vi "rsscope_core_global.vi"() -> ()   [LabVIEW 2014]
doc: "This Global variable contains driver's:\n- Attributes\n- Range Tables\n- Repeated Capabilities"
uses:
  rsidr_core.llb/type_Input_Format_Attribute.ctl
  rsidr_core.llb/rsscope_rsidr_core.lvlib
  rsidr_core.llb/type_Input_Format_RangeTable.ctl
  rsidr_core.llb/type_Input_Format_RepCap.ctl
panel:
  in  "Repeated Capabilities":T1[](array[typedef])=[{"repCapName"="Channel", "indetifiers"=["CH1", "CH2", "CH3", "CH4", "CHExt"], "cmdValues"=["1", "2", "3", "4", "5"]}, {"repCapName"="Waveform", "indetifiers"=["W0", "W1", "W2", "W3"], "cmdValues"=["1", "1", "2", "3"]}, {"repCapName"="Trigger", "indetifiers"=["TrigA", "TrigB", "TrigR"], "cmdValues"=["1", "2", "3"]}, {"repCapName"="Cursor", "indetifiers"=["C1", "C2", "C3", "C4"], "cmdValues"=["1", "2", "3", "4"]}, {"repCapName"="CPosition", "indetifiers"=["P1", "P2"], "cmdValues"=["1", "2"]}, {"repCapName"="TriggerSource", "indetifiers"=["TsCH1", "TsCH2", "TsCH3", "TsCH4", "TsExt", "TsLine", "TsZ1V1", "TsZ1V2", "TsZ1V3", "TsZ1V4", "TsZ1I1", "TsZ1I2", "TsZ1I3", "TsZ1I4", "TsZ2V1", "TsZ2V2", "TsZ2V3", "TsZ2V4", "TsZ2I1", "TsZ2I2", "TsZ2I3", "TsZ2I4", "TsDiff1", "TsDiff2", "TsCommon1", "TsCommon2"], "cmdValues"=["1", "2", "3", "4", "5", "10", "12", "13", "14", "15", "16", "17", "18", "19", "20", "21", "22", "23", "24", "25", "26", "27", "28", "29", "30", "31"]}, {"repCapName"="TriggerType", "indetifiers"=["Edge", "Width", "Runt", "Glitch", "Window", "Timeout", "Interval", "Slew", "Data2Clock", "Pattern", "External", "T11", "T12", "NFC", "TV", "CDR"], "cmdValues"=["1", "3", "4", "2", "5", "6", "7", "8", "9", "10", "11", "12", "14", "15", "16", "17"]}, {"repCapName"="Measurement", "indetifiers"=["Meas1", "Meas2", "Meas3", "Meas4", "Meas5", "Meas6", "Meas7", "Meas8", "Meas9", "Meas10"], "cmdValues"=["1", "2", "3", "4", "5", "6", "7", "8", "9", "10"]}, {"repCapName"="AmptMeasurementType", "indetifiers"=["Ampt1", "Ampt2", "Ampt3", "Ampt4", "Ampt5", "Ampt6", "Ampt7", "Ampt8", "Ampt9", "Ampt10", "Ampt11", "Ampt12", "Ampt13", "Ampt14", "Ampt15", "Ampt16", "Ampt17", "Ampt18", "Ampt19", "Ampt20", "Ampt21", "Ampt22", "Ampt23", "Ampt24", "Ampt25", "Ampt26", "Ampt27", "Ampt28", "Ampt29", "Ampt30", "Ampt47", "Ampt31", "Ampt32", "Ampt35", "Ampt36", "Ampt33", "Ampt34", "Ampt46", "Ampt48", "Ampt49"], "cmdValues"=["1", "2", "3", "4", "5", "6", "7", "8", "9", "10", "11", "12", "13", "14", "15", "16", "17", "18", "19", "20", "21", "22", "23", "24", "25", "26", "27", "28", "29", "30", "47", "31", "32", "35", "36", "33", "34", "46", "48", "49"]}, {"repCapName"="EyeMeasurementType", "indetifiers"=["Eye1", "Eye2", "Eye3", "Eye4", "Eye5", "Eye6", "Eye7", "Eye8", "Eye9", "Eye10", "Eye11", "Eye12", "Eye13", "Eye14", "Eye15", "Eye16", "Eye17", "Eye18", "Eye19", "Eye20", "Eye21", "Eye22", "Eye23", "Eye24", "Eye25", "Eye26", "Eye27", "Eye28", "Eye29", "Eye30"], "cmdValues"=["1", "2", "3", "4", "5", "6", "7", "8", "9", "10", "11", "12", "13", "14", "15", "16", "17", "18", "19", "20", "21", "22", "23", "24", "25", "26", "27", "28", "29", "30"]}, {"repCapName"="HistogramMeasurementType", "indetifiers"=["Hist1", "Hist2", "Hist3", "Hist4", "Hist5", "Hist6", "Hist7", "Hist8", "Hist9", "Hist10", "Hist11", "Hist12", "Hist13", "Hist14", "Hist15", "Hist16", "Hist17", "Hist18"], "cmdValues"=["1", "2", "3", "4", "5", "6", "7", "8", "9", "10", "11", "12", "13", "14", "15", "16", "17", "18"]}, {"repCapName"="SpectrumMeasurementType", "indetifiers"=["Spec1", "Spec2", "Spec3", "Spec4", "Spec5", "Spec6", "Spec7", "Spec8", "Spec9", "Spec10", "Spec11", "Spec12"], "cmdValues"=["1", "2", "3", "4", "9", "10", "7", "8", "11", "12", "13", "14"]}, {"repCapName"="Math", "indetifiers"=["M1", "M2", "M3", "M4", "M5", "M6", "M7", "M8"], "cmdValues"=["1", "2", "3", "4", "5", "6", "7", "8"]}, {"repCapName"="WfmSuffix", "indetifiers"=["WfmNone", "WfmC1W1", "WfmC1W2", "WfmC1W3", "WfmC2W1", "WfmC2W2", "WfmC2W3", "WfmC3W1", "WfmC3W2", "WfmC3W3", "WfmC4W1", "WfmC4W2", "WfmC4W3", "WfmMath1", "WfmMath2", "WfmMath3", "WfmMath4", "WfmRef1", "WfmRef2", "WfmRef3", "WfmRef4", "WfmXY1", "WfmXY2", "WfmXY3", "WfmXY4", "WfmMeas1", "WfmMeas2", "WfmMeas3", "WfmMeas4", "WfmMeas5", "WfmMeas6", "WfmMeas7", "WfmMeas8", "WfmSbus1", "WfmSbus2", "WfmSbus3", "WfmSbus4", "WfmD0", "WfmD1", "WfmD2", "WfmD3", "WfmD4", "WfmD5", "WfmD6", "WfmD7", "WfmD8", "WfmD9", "WfmD10", "WfmD11", "WfmD12", "WfmD13", "WfmD14", "WfmD15", "WfmMSO1", "WfmMSO2", "WfmMSO3", "WfmMSO4", "WfmTRK1", "WfmTRK2", "WfmTRK3", "WfmTRK4", "WfmTRK5", "WfmTRK6", "WfmTRK7", "WfmTRK8", "WfmSpectrum1", "WfmSpectrum2", "WfmSpectrum3", "WfmSpectrum4", "WfmSG1TL1", "WfmSG1TL2", "WfmSG2TL1", "WfmSG2TL2", "WfmSG3TL1", "WfmSG3TL2", "WfmSG4TL1", "WfmSG4TL2", "WfmEye1", "WfmEye2", "WfmEye3", "WfmEye4", "WfmZ1V1", "WfmZ1V2", "WfmZ1V3", "WfmZ1V4", "WfmZ1I1", "WfmZ1I2", "WfmZ1I3", "WfmZ1I4", "WfmZ2V1", "WfmZ2V2", "WfmZ2V3", "WfmZ2V4", "WfmZ2I1", "WfmZ2I2", "WfmZ2I3", "WfmZ2I4", "WfmDiff1", "WfmDiff2", "WfmCommon1", "WfmCommon2", "WfmTDRZ", "WfmTDRH", "WfmTDRR", "WfmMath5", "WfmMath6", "WfmMath7", "WfmMath8", "WfmSpectrum5", "WfmSpectrum6", "WfmSpectrum7", "WfmSpectrum8", "WfmSG5TL1", "WfmSG5TL2", "WfmSG6TL1", "WfmSG6TL2", "WfmSG7TL1", "WfmSG7TL2", "WfmSG8TL1", "WfmSG8TL2", "WfmHP1", "WfmHP2", "WfmHP3", "WfmHP4", "WfmHP5", "WfmHP6", "WfmHP7", "WfmHP8", "WfmHP9", "WfmHP10", "WfmBathtub1", "WfmBathMeas1", "WfmStepResp1", "WfmSRHist1", "WfmSDHist1", "WfmTJHist1", "WfmDJHist1", "WfmDDJHist1", "WfmPJHist1", "WfmRJOHist1", "WfmSRTrack1", "WfmTJTrack1", "WfmDJTrack1", "WfmDDJTrack1", "WfmPJTrack1", "WfmRJTrack1", "WfmTJSpectrum1", "WfmDDJSpectrum1", "WfmPJSpectrum1", "WfmRJSpectrum1", "WfmSEye1", "WfmBathtub2", "WfmBathMeas2", "WfmStepResp2", "WfmSRHist2", "WfmSDHist2", "WfmTJHist2", "WfmDJHist2", "WfmDDJHist2", "WfmPJHist2", "WfmRJOHist2", "WfmSRTrack2", "WfmSDTrack2", "WfmTJTrack2", "WfmDDJTrack2", "WfmPJTrack2", "WfmRJTrack2", "WfmTJSpectrum2", "WfmDDJSpectrum2", "WfmPJSpectrum2", "WfmRJSpectrum2", "WfmSEye2", "WfmNBathtub1", "WfmNBathMeas1", "WfmTNHist1", "WfmDNHist1", "WfmDDNHist1", "WfmPNHist1", "WfmRNOTrack1", "WfmTNTrack1", "WfmDDNTrack1", "WfmPNTrack1", "WfmRNTrack1", "WfmTNSpectrum1", "WfmDDNSpectrum1", "WfmPNSpectrum1", "WfmRNSpectrum1", "WfmNBathtub2", "WfmNBathMeas2", "WfmTNHist2", "WfmDNHist2", "WfmDDNHist2", "WfmPNHist2", "WfmRNOHist2", "WfmTNTrack2", "WfmDDNTrack2", "WfmPNTrack2", "WfmRNTrack2", "WfmTNSpectrum2", "WfmDDNSpectrum2", "WfmPNSpectrum2", "WfmRNSpectrum2", "WfmPJDHist1", "WfmBUJHist1", "WfmRJHist1", "WfmPJDTrack1", "WfmPJDSpectrum1", "WfmPJDHist2", "WfmBUJHist2", "WfmRJHist2", "WfmPJDTrack2", "WfmPJDSpectrum2", "WfmPNDHist1", "WfmBUNHist1", "WfmRNHist1", "WfmPNDTrack1", "WfmPNDSpectrum1", "WfmPNDHist2", "WfmBUNHist2", "WfmRNHist2", "WfmPNDTrack2", "WfmPNDSpectrum2"], "cmdValues"=["1", "2", "3", "4", "5", "6", "7", "8", "9", "10", "11", "12", "13", "14", "15", "16", "17", "18", "19", "20", "21", "22", "23", "24", "25", "26", "27", "28", "29", "30", "31", "32", "33", "36", "37", "38", "39", "40", "41", "42", "43", "44", "45", "46", "47", "48", "49", "50", "51", "52", "53", "54", "55", "56", "57", "58", "59", "61", "62", "63", "64", "65", "66", "67", "68", "72", "73", "74", "75", "76", "77", "78", "79", "80", "81", "82", "83", "84", "85", "86", "87", "88", "89", "90", "91", "92", "93", "94", "95", "96", "97", "98", "99", "100", "101", "102", "103", "108", "109", "110", "111", "112", "113", "114", "115", "116", "117", "118", "119", "120", "121", "122", "123", "124", "125", "126", "127", "128", "129", "130", "131", "132", "133", "134", "135", "136", "137", "138", "139", "140", "142", "143", "144", "145", "146", "147", "148", "149", "150", "151", "152", "154", "155", "156", "157", "158", "159", "160", "161", "162", "163", "165", "166", "167", "168", "169", "170", "171", "172", "173", "174", "175", "176", "177", "179", "180", "181", "182", "183", "184", "185", "186", "187", "188", "189", "190", "191", "192", "193", "194", "196", "197", "198", "199", "200", "201", "202", "203", "204", "205", "206", "207", "208", "209", "210", "212", "213", "214", "215", "216", "217", "218", "219", "220", "221", "222", "223", "224", "225", "226", "227", "228", "229", "230", "231", "232", "233", "234", "235", "236", "237", "238"]}, {"repCapName"="ReferenceWfm", "indetifiers"=["RW1", "RW2", "RW3", "RW4"], "cmdValues"=["1", "2", "3", "4"]}, {"repCapName"="SerialBus", "indetifiers"=["SB1", "SB2", "SB3", "SB4"], "cmdValues"=["1", "2", "3", "4"]}, {"repCapName"="Destination", "indetifiers"=["DE1", "DE2"], "cmdValues"=["1", "2"]}, {"repCapName"="XYDiagram", "indetifiers"=["XY1", "XY2", "XY3", "XY4"], "cmdValues"=["1", "2", "3", "4"]}, {"repCapName"="CANTimeSeg", "indetifiers"=["TS1", "TS2"], "cmdValues"=["1", "2"]}, {"repCapName"="ORSlot", "indetifiers"=["ORSlot1", "ORSlot2", "ORSlot3", "ORSlot4"], "cmdValues"=["1", "2", "3", "4"]}, {"repCapName"="SourceNumber", "indetifiers"=["SN1", "SN2", "SN3", "SN4"], "cmdValues"=["1", "2", "3", "4"]}, {"repCapName"="Line", "indetifiers"=["Data", "Enable"], "cmdValues"=["1", "2"]}, {"repCapName"="DigitalChannel", "indetifiers"=["D0", "D1", "D2", "D3", "D4", "D5", "D6", "D7", "D8", "D9", "D10", "D11", "D12", "D13", "D14", "D15"], "cmdValues"=["0", "1", "2", "3", "4", "5", "6", "7", "8", "9", "10", "11", "12", "13", "14", "15"]}, {"repCapName"="ChannelGroup", "indetifiers"=["CG1", "CG2", "CG3", "CG4"], "cmdValues"=["1", "2", "3", "4"]}, {"repCapName"="ConditionNumber", "indetifiers"=["Con1", "Con2", "Con3", "Con4"], "cmdValues"=["1", "2", "3", "4"]}, {"repCapName"="TDMChannel", "indetifiers"=["TDM1", "TDM2", "TDM3", "TDM4", "TDM5", "TDM6", "TDM7", "TDM8"], "cmdValues"=["1", "2", "3", "4", "5", "6", "7", "8"]}, {"repCapName"="JitterMeasurementType", "indetifiers"=["Jitt1", "Jitt2", "Jitt3", "Jitt4", "Jitt5", "Jitt6", "Jitt7", "Jitt8", "Jitt9"], "cmdValues"=["37", "38", "39", "40", "41", "42", "43", "44", "45"]}, {"repCapName"="SW", "indetifiers"=["SW1", "SW2"], "cmdValues"=["1", "2"]}, {"repCapName"="Gate", "indetifiers"=["Gate1", "Gate2", "Gate3", "Gate4", "Gate5"], "cmdValues"=["1", "2", "3", "4", "5"]}, {"repCapName"="ResultNumber", "indetifiers"=["Res1", "Res2", "Res3", "Res4", "Res5", "Res6", "Res7", "Res8"], "cmdValues"=["1", "2", "3", "4", "5", "6", "7", "8"]}, {"repCapName"="ResultHarmonics", "indetifiers"=["Harm1", "Harm2", "Harm3", "Harm4", "Harm5", "Harm6", "Harm7", "Harm8", "Harm9", "Harm10", "Harm11", "Harm12", "Harm13", "Harm14", "Harm15", "Harm16", "Harm17", "Harm18", "Harm19", "Harm20", "Harm21", "Harm22", "Harm23", "Harm24", "Harm25", "Harm26", "Harm27", "Harm28", "Harm29", "Harm30", "Harm31", "Harm32", "Harm33", "Harm34", "Harm35", "Harm36", "Harm37", "Harm38", "Harm39", "Herm40"], "cmdValues"=["1", "2", "3", "4", "5", "6", "7", "8", "9", "10", "11", "12", "13", "14", "15", "16", "17", "18", "19", "20", "21", "22", "23", "24", "25", "26", "27", "28", "29", "30", "31", "32", "33", "34", "35", "36", "37", "38", "39", "40"]}, {"repCapName"="Timeline", "indetifiers"=["TL1", "TL2"], "cmdValues"=["1", "2"]}, {"repCapName"="Math2", "indetifiers"=["M21", "M22", "M23", "M24", "M25", "M26", "M27", "M28"], "cmdValues"=["1", "2", "3", "4", "5", "6", "7", "8"]}, {"repCapName"="WaveformGenerator", "indetifiers"=["WG1", "WG2"], "cmdValues"=["1", "2"]}, {"repCapName"="FieldNumber", "indetifiers"=["Field1", "Field2", "Field3", "Field4", "Field5", "Field6", "Field7", "Field8", "Field9", "Field10", "Field11", "Field12", "Field13", "Field14", "Field15", "Field16", "Field17", "Field18", "Field19", "Field20"], "cmdValues"=["1", "2", "3", "4", "5", "6", "7", "8", "9", "10", "11", "12", "13", "14", "15", "16", "17", "18", "19", "20"]}, {"repCapName"="ZVCZ", "indetifiers"=["ZVCZ1", "ZVCZ2"], "cmdValues"=["1", "2"]}, {"repCapName"="ZVCV", "indetifiers"=["ZVCV1", "ZVCV2", "ZVCV3", "ZVCV4"], "cmdValues"=["1", "2", "3", "4"]}, {"repCapName"="ZVCI", "indetifiers"=["ZVCI1", "ZVCI2", "ZVCI3", "ZVCI4"], "cmdValues"=["1", "2", "3", "4"]}, {"repCapName"="EyeDiagram", "indetifiers"=["ED1", "ED2", "ED3", "ED4"], "cmdValues"=["1", "2", "3", "4"]}, {"repCapName"="ComplexCondition", "indetifiers"=["Complex1", "Complex2", "Complex3", "Complex4"], "cmdValues"=["1", "2", "3", "4"]}, {"repCapName"="EbTbSymbol", "indetifiers"=["EbTb1", "EbTb2", "EbTb3", "EbTb4", "EbTb5", "EbTb6", "EbTb7", "EbTb8", "EbTb9", "EbTb10", "EbTb11", "EbTb12", "EbTb13", "EbTb14", "EbTb15", "EbTb16"], "cmdValues"=["1", "2", "3", "4", "5", "6", "7", "8", "9", "10", "11", "12", "13", "14", "15", "16"]}, {"repCapName"="CoupledChannel", "indetifiers"=["CplCH1", "CplCH2", "CplCH3", "CplCH4"], "cmdValues"=["1", "2", "3", "4"]}, {"repCapName"="DifferentialSignal", "indetifiers"=["Diff1", "Diff2"], "cmdValues"=["1", "2"]}, {"repCapName"="DecodeTable", "indetifiers"=["DecTbl1", "DecTbl2", "DecTbl3", "DecTbl4", "DecTbl5"], "cmdValues"=["1", "2", "3", "4", "5"]}, {"repCapName"="TDRTDTSignal", "indetifiers"=["Imped", "RCoeff", "PResp"], "cmdValues"=["1", "2", "3"]}, {"repCapName"="AdvJitterMeas", "indetifiers"=["JA1", "JA2"], "cmdValues"=["1", "2"]}, {"repCapName"="AdvJitterComponent", "indetifiers"=["f_symb", "T_symb", "EC", "TJ_BER", "RJ", "DDirac", "TJ", "DJ", "DDJ", "DCD", "PJ", "ISI"], "cmdValues"=["1", "2", "3", "4", "5", "6", "7", "8", "9", "10", "11", "12"]}, {"repCapName"="AdvJitterPeriodicComponent", "indetifiers"=["Periodic1", "Periodic2", "Periodic3", "Periodic4", "Periodic5", "Periodic6", "Periodic7", "Periodic8", "Periodic9", "Periodic10"], "cmdValues"=["1", "2", "3", "4", "5", "6", "7", "8", "9", "10"]}, {"repCapName"="ArithmeticParameter", "indetifiers"=["ArithmeticParm1", "ArithmeticParm2"], "cmdValues"=["1", "2"]}]
  in  "Range Tables":T2[](array[typedef])=[{"Type"=0, "Name"="rsscope_rngHorzScale", "Entries"=[{"Name"="", "Value 1"=2.5e-11, "Value 2"=10000.0, "Command"=""}]}, {"Type"=0, "Name"="rsscope_rngHorzAcquisitionTime", "Entries"=[{"Name"="", "Value 1"=2.5e-10, "Value 2"=100000.0, "Command"=""}]}, {"Type"=0, "Name"="rsscope_rngHorzReference", "Entries"=[{"Name"="", "Value 1"=0.0, "Value 2"=100.0, "Command"=""}]}, {"Type"=2, "Name"="rsscope_rngSampleMode", "Entries"=[{"Name"="Real Time", "Value 1"=0.0, "Value 2"=0.0, "Command"="RTIM"}, {"Name"="Equivalent Time", "Value 1"=1.0, "Value 2"=0.0, "Command"="ETIM"}, {"Name"="Interpolated Time", "Value 1"=2.0, "Value 2"=0.0, "Command"="ITIM"}]}, {"Type"=2, "Name"="rsscope_rngWaveformArithmetics", "Entries"=[{"Name"="Off", "Value 1"=0.0, "Value 2"=0.0, "Command"="OFF"}, {"Name"="Envelope", "Value 1"=1.0, "Value 2"=0.0, "Command"="ENV"}, {"Name"="Average", "Value 1"=2.0, "Value 2"=0.0, "Command"="AVER"}, {"Name"="RMS", "Value 1"=3.0, "Value 2"=0.0, "Command"="RMS"}, {"Name"="Min Hold", "Value 1"=4.0, "Value 2"=0.0, "Command"="MINH"}, {"Name"="Max Hold", "Value 1"=5.0, "Value 2"=0.0, "Command"="MAXH"}]}, {"Type"=2, "Name"="rsscope_rngVerticalCoupling", "Entries"=[{"Name"="AC", "Value 1"=0.0, "Value 2"=0.0, "Command"="AC"}, {"Name"="DC 50 Ohm", "Value 1"=1.0, "Value 2"=0.0, "Command"="DC"}, {"Name"="DC 1 MOhm", "Value 1"=2.0, "Value 2"=0.0, "Command"="DCL"}]}, {"Type"=0, "Name"="rsscope_rngVerticalOffset", "Entries"=[{"Name"="", "Value 1"=-5.0, "Value 2"=5.0, "Command"=""}]}, {"Type"=2, "Name"="rsscope_rngChannelBWLimit", "Entries"=[{"Name"="Full", "Value 1"=0.0, "Value 2"=0.0, "Command"="FULL"}, {"Name"="800 MHz", "Value 1"=1.0, "Value 2"=0.0, "Command"="B800"}, {"Name"="200 MHz", "Value 1"=2.0, "Value 2"=0.0, "Command"="B200"}, {"Name"="20 MHz", "Value 1"=3.0, "Value 2"=0.0, "Command"="B20"}]}, {"Type"=2, "Name"="rsscope_rngTriggerMode", "Entries"=[{"Name"="Normal", "Value 1"=0.0, "Value 2"=0.0, "Command"="NORM"}, {"Name"="Auto", "Value 1"=1.0, "Value 2"=0.0, "Command"="AUTO"}, {"Name"="Free Run", "Value 1"=2.0, "Value 2"=0.0, "Command"="FRE"}]}, {"Type"=2, "Name"="rsscope_rngTriggerSource", "Entries"=[{"Name"="Channel 1", "Value 1"=1.0, "Value 2"=0.0, "Command"="CHAN1"}, {"Name"="Channel 2", "Value 1"=2.0, "Value 2"=0.0, "Command"="CHAN2"}, {"Name"="Channel 3", "Value 1"=3.0, "Value 2"=0.0, "Command"="CHAN3"}, {"Name"="Channel 4", "Value 1"=4.0, "Value 2"=0.0, "Command"="CHAN4"}, {"Name"="External", "Value 1"=5.0, "Value 2"=0.0, "Command"="EXT"}, {"Name"="Serial Bus", "Value 1"=6.0, "Value 2"=0.0, "Command"="SBUS"}, {"Name"="Line", "Value 1"=7.0, "Value 2"=0.0, "Command"="LINE"}, {"Name"="Digital Channel 0", "Value 1"=8.0, "Value 2"=0.0, "Command"="D0"}, {"Name"="Digital Channel 1", "Value 1"=9.0, "Value 2"=0.0, "Command"="D1"}, {"Name"="Digital Channel 2", "Value 1"=10.0, "Value 2"=0.0, "Command"="D2"}, {"Name"="Digital Channel 3", "Value 1"=11.0, "Value 2"=0.0, "Command"="D3"}, {"Name"="Digital Channel 4", "Value 1"=12.0, "Value 2"=0.0, "Command"="D4"}, {"Name"="Digital Channel 5", "Value 1"=13.0, "Value 2"=0.0, "Command"="D5"}, {"Name"="Digital Channel 6", "Value 1"=14.0, "Value 2"=0.0, "Command"="D6"}, {"Name"="Digital Channel 7", "Value 1"=15.0, "Value 2"=0.0, "Command"="D7"}, {"Name"="Digital Channel 8", "Value 1"=16.0, "Value 2"=0.0, "Command"="D8"}, {"Name"="Digital Channel 9", "Value 1"=17.0, "Value 2"=0.0, "Command"="D9"}, {"Name"="Digital Channel 10", "Value 1"=18.0, "Value 2"=0.0, "Command"="D10"}, {"Name"="Digital Channel 11", "Value 1"=19.0, "Value 2"=0.0, "Command"="D11"}, {"Name"="Digital Channel 12", "Value 1"=20.0, "Value 2"=0.0, "Command"="D12"}, {"Name"="Digital Channel 13", "Value 1"=21.0, "Value 2"=0.0, "Command"="D13"}, {"Name"="Digital Channel 14", "Value 1"=22.0, "Value 2"=0.0, "Command"="D14"}, {"Name"="Digital Channel 15", "Value 1"=23.0, "Value 2"=0.0, "Command"="D15"}, {"Name"="Logic", "Value 1"=24.0, "Value 2"=0.0, "Command"="LOG"}, {"Name"="Parallel Bus 1", "Value 1"=25.0, "Value 2"=0.0, "Command"="MSOB1"}, {"Name"="Parallel Bus 2", "Value 1"=26.0, "Value 2"=0.0, "Command"="MSOB2"}, {"Name"="Parallel Bus 3", "Value 1"=27.0, "Value 2"=0.0, "Command"="MSOB3"}, {"Name"="Parallel Bus 4", "Value 1"=28.0, "Value 2"=0.0, "Command"="MSOB4"}, {"Name"="Probe 1 Voltage 1", "Value 1"=29.0, "Value 2"=0.0, "Command"="Z1V1"}, {"Name"="Probe 1 Voltage 2", "Value 1"=30.0, "Value 2"=0.0, "Command"="Z1V2"}, {"Name"="Probe 1 Voltage 3", "Value 1"=31.0, "Value 2"=0.0, "Command"="Z1V3"}, {"Name"="Probe 1 Voltage 4", "Value 1"=32.0, "Value 2"=0.0, "Command"="Z1V4"}, {"Name"="Probe 1 Current 1", "Value 1"=33.0, "Value 2"=0.0, "Command"="Z1I1"}, {"Name"="Probe 1 Current 2", "Value 1"=34.0, "Value 2"=0.0, "Command"="Z1I2"}, {"Name"="Probe 1 Current 3", "Value 1"=35.0, "Value 2"=0.0, "Command"="Z1I3"}, {"Name"="Probe 1 Current 4", "Value 1"=36.0, "Value 2"=0.0, "Command"="Z1I4"}, {"Name"="Probe 2 Voltage 1", "Value 1"=37.0, "Value 2"=0.0, "Command"="Z2V1"}, {"Name"="Probe 2 Voltage 2", "Value 1"=38.0, "Value 2"=0.0, "Command"="Z2V2"}, {"Name"="Probe 2 Voltage 3", "Value 1"=39.0, "Value 2"=0.0, "Command"="Z2V3"}, {"Name"="Probe 2 Voltage 4", "Value 1"=40.0, "Value 2"=0.0, "Command"="Z2V4"}, {"Name"="Probe 2 Current 1", "Value 1"=41.0, "Value 2"=0.0, "Command"="Z2I1"}, {"Name"="Probe 2 Current 2", "Value 1"=42.0, "Value 2"=0.0, "Command"="Z2I2"}, {"Name"="Probe 2 Current 3", "Value 1"=43.0, "Value 2"=0.0, "Command"="Z2I3"}, {"Name"="Probe 2 Current 4", "Value 1"=44.0, "Value 2"=0.0, "Command"="Z2I4"}, {"Name"="Diff1", "Value 1"=45.0, "Value 2"=0.0, "Command"="DIFF1"}, {"Name"="Diff2", "Value 1"=46.0, "Value 2"=0.0, "Command"="DIFF2"}, {"Name"="Common1", "Value 1"=47.0, "Value 2"=0.0, "Command"="COMMON1"}, {"Name"="Common2", "Value 1"=48.0, "Value 2"=0.0, "Command"="COMMON2"}]}, ...(904 in all)] {"Type" items=["Range", "Coerced", "Discrete"]}
  in  "Attributes":T3[](array[typedef])=[{"Level"=1, "Class Only"=TRUE, "Identifier"="", "Descriptive Name"="Acquisition", "Data Type"=0, "Command"="", "Access"=0, "Range Table"="", "Read Callback"="", "Write Callback"="", "Supported Models"="", "Instrument Options"="", "Flags"=0, "Help"="This class contains attributes that configure the acquisition subsystem."}, {"Level"=2, "Class Only"=FALSE, "Identifier"="RSSCOPE_ATTR_INTERPOLATION", "Descriptive Name"="Interpolation", "Data Type"=0, "Command"="ACQ:INT", "Access"=2, "Range Table"="rsscope_rngInterpolation", "Read Callback"="", "Write Callback"="", "Supported Models"="", "Instrument Options"="", "Flags"=0, "Help"="Selects the interpolation method if ACQuire:MODE ITIMe (interpolated time) is set for enhancement.\n\nAvailable Repeated Capabilities:\nNone\n\nRemote-control command(s):\nACQuire:INTerpolate"}, {"Level"=2, "Class Only"=FALSE, "Identifier"="RSSCOPE_ATTR_NUM_AVERAGES", "Descriptive Name"="Number of Averages", "Data Type"=0, "Command"="ACQ:COUN", "Access"=2, "Range Table"="", "Read Callback"="", "Write Callback"="", "Supported Models"="", "Instrument Options"="", "Flags"=0, "Help"="Defines the &apos;Average count&apos; that has a double effect:\n- it defines the number of waveforms used to calculate the average waveform, and\n- it sets the number of waveforms acquired with RUNSingle.\n\nAvailable Repeated Capabilities:\nNone\n\nRemote-control command(s):\nACQuire:COUNt"}, {"Level"=2, "Class Only"=FALSE, "Identifier"="RSSCOPE_ATTR_SAMPLE_MODE", "Descriptive Name"="Sample Mode", "Data Type"=0, "Command"="ACQ:MODE", "Access"=2, "Range Table"="rsscope_rngSampleMode", "Read Callback"="", "Write Callback"="", "Supported Models"="", "Instrument Options"="", "Flags"=0, "Help"="Selects the method of adding waveform points to the samples of the ADC in order to fill the record length.\n\nAvailable Repeated Capabilities:\nNone\n\nRemote-control command(s):\nACQuire:MODE"}, {"Level"=2, "Class Only"=FALSE, "Identifier"="RSSCOPE_ATTR_HORZ_RECORD_SELECTION", "Descriptive Name"="Horizontal Record Selection", "Data Type"=0, "Command"="ACQ:POIN:AUTO", "Access"=2, "Range Table"="rsscope_rngHorzRecordSelection", "Read Callback"="", "Write Callback"="", "Supported Models"="", "Instrument Options"="", "Flags"=0, "Help"="Selection to change either the resolution or the record length. The other value remains constant and cannot be changed.\n\nAvailable Repeated Capabilities:\nNone\n\nRemote-control command(s):\nACQuire:POINts:AUTO"}, {"Level"=2, "Class Only"=FALSE, "Identifier"="RSSCOPE_ATTR_ACQUISITION_AUTO_ADJUSTMENT", "Descriptive Name"="Acquisition Auto Adjustment", "Data Type"=3, "Command"="ACQ:POIN:AADJ", "Access"=2, "Range Table"="", "Read Callback"="", "Write Callback"="", "Supported Models"="", "Instrument Options"="", "Flags"=0, "Help"="Prevents undersampling and ensures a sufficient resolution to acquire the correct waveform if the time scale is changed. The setting takes effect if the changed parameter - resolution or record length - reaches a limit.\n\nAvailable Repeated Capabilities:\nNone\n\nRemote-control command(s):\nACQuire:POINts:AADJust"}, {"Level"=2, "Class Only"=FALSE, "Identifier"="RSSCOPE_ATTR_HORZ_TIME_PER_RECORD", "Descriptive Name"="Horizontal Time Per Record", "Data Type"=1, "Command"="TIM:RANG", "Access"=2, "Range Table"="rsscope_rngHorzAcquisitionTime", "Read Callback"="", "Write Callback"="", "Supported Models"="", "Instrument Options"="", "Flags"=0, "Help"="Defines the time of one acquisition, that is the time across the 10 divisions of the diagram: Horizontal Scale *10.\n\nAvailable Repeated Capabilities:\nNone\n\nRemote-control command(s):\nTIMebase:RANGe"}, {"Level"=2, "Class Only"=FALSE, "Identifier"="RSSCOPE_ATTR_HORZ_RECORD_LENGTH", "Descriptive Name"="Horizontal Record Length", "Data Type"=0, "Command"="ACQ:POIN", "Access"=2, "Range Table"="rsscope_rngHorzRecordLength", "Read Callback"="", "Write Callback"="", "Supported Models"="", "Instrument Options"="", "Flags"=0, "Help"="Indicates the record length, the number of recorded waveform points that build the waveform across the acquisition time.\n\nAvailable Repeated Capabilities:\nNone\n\nRemote-control command(s):\nACQuire:POINts[:VALue]"}, {"Level"=2, "Class Only"=FALSE, "Identifier"="RSSCOPE_ATTR_HORZ_RECORD_LENGTH_LIMIT", "Descriptive Name"="Horizontal Record Length Limit", "Data Type"=0, "Command"="ACQ:POIN:MAX", "Access"=2, "Range Table"="rsscope_rngHorzRecordLength", "Read Callback"="", "Write Callback"="", "Supported Models"="", "Instrument Options"="", "Flags"=0, "Help"="This attribute configures the limit for the record length to prevent very large records.If you increase the time scale, the resolution remains constant and the record length increases until the limit is reached. Further increase of the time scale changes the resolution and keeps the record length limit.\n\nNote: This value is only available if &apos;Auto adjustment&apos; is ON and a constant resolution is selected.\n\nAvailable Repeated Capabilities:\nNone\n\nRemote-control command(s):\nACQuire:POINts:MAXimum"}, {"Level"=2, "Class Only"=FALSE, "Identifier"="RSSCOPE_ATTR_HORZ_SCALE", "Descriptive Name"="Horizontal Scale", "Data Type"=1, "Command"="TIM:SCAL", "Access"=2, "Range Table"="rsscope_rngHorzScale", "Read Callback"="", "Write Callback"="", "Supported Models"="", "Instrument Options"="", "Flags"=0, "Help"="Sets the horizontal scale - the time per division on the x-axis - for all channel and math waveforms.\nThe setting accuracy depends on the current resolution (sample rate) and the setting for resolution enhancement:\n- In interpolated time mode if sample rate > ADC sample rate: Any value for the horizontal scale can be set due to the interpolation factor.\n- In real time mode and equivalent time mode for all sample rates; and in interpolated time mode if sample rate < ADC sample rate: The resolution is an integer multiple of the ADC sample rate.\n\nAvailable Repeated Capabilities:\nNone\n\nRemote-control command(s):\nTIMebase:SCALe"}, {"Level"=2, "Class Only"=FALSE, "Identifier"="RSSCOPE_ATTR_ZVC_RECORD_LENGTH", "Descriptive Name"="ZVC Record Length", "Data Type"=0, "Command"="ACQ:POIN:ZVAL?", "Access"=0, "Range Table"="", "Read Callback"="", "Write Callback"="", "Supported Models"="", "Instrument Options"="", "Flags"=0, "Help"="Returns the current record length used by the R&S RT-ZVC multi-channel high accuracy power probe channel.\n\nAvailable Repeated Capabilities:\nNone\n\nRemote-control command(s):\nACQuire:POINts:ZVALue?"}, {"Level"=2, "Class Only"=FALSE, "Identifier"="RSSCOPE_ATTR_ZVC_CURRENT_RESOLUTION", "Descriptive Name"="ZVC Current Resolution", "Data Type"=1, "Command"="ACQ:ZRES?", "Access"=0, "Range Table"="", "Read Callback"="", "Write Callback"="", "Supported Models"="", "Instrument Options"="", "Flags"=0, "Help"="Returns the current resolution of the R&S RT-ZVC multi-channel high accuracy power probe channel.\n\nAvailable Repeated Capabilities:\nNone\n\nRemote-control command(s):\nACQuire:ZRESolution?"}, {"Level"=2, "Class Only"=FALSE, "Identifier"="RSSCOPE_ATTR_ACQUSITION_START_TIME", "Descriptive Name"="Acqusition Start Time", "Data Type"=1, "Command"="TIM:HOR:POS", "Access"=2, "Range Table"="", "Read Callback"="", "Write Callback"="", "Supported Models"="", "Instrument Options"="", "Flags"=0, "Help"="Defines the trigger offset - the time interval between trigger point and reference point to analyze the signal some time before or after the trigger event.\n\nAvailable Repeated Capabilities:\nNone\n\nRemote-control command(s):\nTIMebase:HORizontal:POSition"}, {"Level"=2, "Class Only"=FALSE, "Identifier"="RSSCOPE_ATTR_NUMBER_OF_ACQUISITIONS", "Descriptive Name"="Number Of Acquisitions", "Data Type"=0, "Command"="ACQ:CURR?", "Access"=0, "Range Table"="", "Read Callback"="", "Write Callback"="", "Supported Models"="", "Instrument Options"="", "Flags"=0, "Help"="Shows the current number of acquisitions that have been acquired.\n\nAvailable Repeated Capabilities:\nNone\n\nRemote-control command(s):\nACQuire:CURRent?"}, {"Level"=2, "Class Only"=FALSE, "Identifier"="RSSCOPE_ATTR_ACQUISITION_RESTRICT_OFFSET", "Descriptive Name"="Acquisition Restrict Offset", "Data Type"=3, "Command"="TRIG:OFFS:LIM", "Access"=2, "Range Table"="", "Read Callback"="", "Write Callback"="", "Supported Models"="", "Instrument Options"="", "Flags"=0, "Help"="Ensures that the trigger occurs within one acquisition cycle.\n\nAvailable Repeated Capabilities:\nNone\n\nRemote-control command(s):\nTRIGger<m>:OFFSet:LIMited"}, {"Level"=2, "Class Only"=FALSE, "Identifier"="RSSCOPE_ATTR_ACQUISITION_SAMPLE_RATE", "Descriptive Name"="Acquisition Sample Rate", "Data Type"=1, "Command"="ACQ:SRR", "Access"=2, "Range Table"="RsScope_rngAcquisitionSampleRate", "Read Callback"="", "Write Callback"="", "Supported Models"="", "Instrument Options"="", "Flags"=0, "Help"="Sets the number of captured waveform points per second. It considers the samples of the ADC, and the reduction of waveform points by decimation.\nIf interpolation is not active, the sample rate is the reciprocal value of the resolution and thus also depends on the acquisition time and the record length.\nIf interpolation is active, the sample rate is limited to the ADC sample rate.\n\nAvailable Repeated Capabilities:\nNone\n\nRemote-control command(s):\nACQuire:SRReal"}, {"Level"=2, "Class Only"=FALSE, "Identifier"="RSSCOPE_ATTR_ACQUISITION_TIME", "Descriptive Name"="Acquisition Time", "Data Type"=1, "Command"="TIM:RACT?", "Access"=0, "Range Table"="", "Read Callback"="", "Write Callback"="", "Supported Models"="", "Instrument Options"="", "Flags"=0, "Help"="Queries the required acquisition time. If FFT gating is used and the resolution BW is set to constant, record length can be extended to acquire the required number of samples. In this case, the required acquisition time differs from the adjusted acquisition time.\n\nAvailable Repeated Capabilities:\nNone\n\nRemote-control command(s):\nTIMebase:RACTime?"}, {"Level"=2, "Class Only"=FALSE, "Identifier"="RSSCOPE_ATTR_HORZ_SAMPLE_RATE", "Descriptive Name"="Horizontal Sample Rate", "Data Type"=1, "Command"="ACQ:SRAT", "Access"=2, "Range Table"="", "Read Callback"="", "Write Callback"="", "Supported Models"="", "Instrument Options"="", "Flags"=0, "Help"="Defines the sample rate, that is the number of recorded waveform samples per second.\n\nAvailable Repeated Capabilities:\nNone\n\nRemote-control command(s):\nACQuire:SRATe"}, {"Level"=2, "Class Only"=FALSE, "Identifier"="RSSCOPE_ATTR_HORZ_ADC_SAMPLE_RATE", "Descriptive Name"="Horizontal ADC Sample Rate", "Data Type"=1, "Command"="ACQ:POIN:ARAT?", "Access"=0, "Range Table"="", "Read Callback"="", "Write Callback"="", "Supported Models"="", "Instrument Options"="", "Flags"=0, "Help"="Retrieves the sample rate of the ADC, that is the number of points that are sampled by the ADC in one second.\n\nAvailable Repeated Capabilities:\nNone\n\nRemote-control command(s):\nACQuire:POINts:ARATe?"}, {"Level"=2, "Class Only"=FALSE, "Identifier"="RSSCOPE_ATTR_AUTOSCALE", "Descriptive Name"="Autoscale", "Data Type"=4, "Command"="AUT", "Access"=1, "Range Table"="", "Read Callback"="", "Write Callback"="", "Supported Models"="", "Instrument Options"="", "Flags"=1, "Help"="Performs an autoset process: analyzes the enabled channel signals, and obtains appropriate horizontal, vertical, and trigger settings to display stable waveforms\n\nAvailable Repeated Capabilities:\nNone\n\nRemote-control command(s):\nAUToscale"}, {"Level"=2, "Class Only"=FALSE, "Identifier"="RSSCOPE_ATTR_HORZ_DIVISIONS", "Descriptive Name"="Horizontal Divisions", "Data Type"=0, "Command"="TIM:DIV?", "Access"=0, "Range Table"="", "Read Callback"="", "Write Callback"="", "Supported Models"="", "Instrument Options"="", "Flags"=0, "Help"="Queries the number of horizontal divisions on the screen. The number cannot be changed.\n\nAvailable Repeated Capabilities:\nNone\n\nRemote-control command(s):\nTIMebase:DIVisions?"}, {"Level"=2, "Class Only"=FALSE, "Identifier"="RSSCOPE_ATTR_HORZ_REFERENCE", "Descriptive Name"="Horizontal Reference", "Data Type"=0, "Command"="TIM:REF", "Access"=2, "Range Table"="rsscope_rngHorzReference", "Read Callback"="", "Write Callback"="", "Supported Models"="", "Instrument Options"="", "Flags"=0, "Help"="Sets the reference point of the time scale in % of the display. The reference point defines which part of the waveform is shown. If the &apos;Trigger offset&apos; is zero, the trigger point matches the reference point.\n\nAvailable Repeated Capabilities:\nNone\n\nRemote-control command(s):\nTIMebase:REFerence"}, {"Level"=2, "Class Only"=FALSE, "Identifier"="RSSCOPE_ATTR_HORZ_RESOLUTION", "Descriptive Name"="Horizontal Resolution", "Data Type"=1, "Command"="ACQ:RES", "Access"=2, "Range Table"="", "Read Callback"="", "Write Callback"="", "Supported Models"="", "Instrument Options"="", "Flags"=0, "Help"="Indicates the time between two waveform points in the record.\n\nAvailable Repeated Capabilities:\nNone\n\nRemote-control command(s):\nACQuire:RESolution"}, {"Level"=2, "Class Only"=FALSE, "Identifier"="RSSCOPE_ATTR_ROLL_MODE_AUTO", "Descriptive Name"="Roll Mode Auto", "Data Type"=0, "Command"="TIM:ROLL:ENAB", "Access"=2, "Range Table"="rsscope_rngRollModeAuto", "Read Callback"="", "Write Callback"="", "Supported Models"="", "Instrument Options"="", "Flags"=0, "Help"="Activates the automatic roll mode.\n\nAvailable Repeated Capabilities:\nNone\n\nRemote-control command(s):\nTIMebase:ROLL:ENABle"}, {"Level"=2, "Class Only"=FALSE, "Identifier"="RSSCOPE_ATTR_ROLL_STATE", "Descriptive Name"="Roll State", "Data Type"=3, "Command"="TIM:ROLL:STAT?", "Access"=0, "Range Table"="", "Read Callback"="", "Write Callback"="", "Supported Models"="", "Instrument Options"="", "Flags"=0, "Help"="Returns the status of the roll mode.\n\nAvailable Repeated Capabilities:\nNone\n\nRemote-control command(s):\nTIMebase:ROLL:STATe?"}, {"Level"=2, "Class Only"=FALSE, "Identifier"="RSSCOPE_ATTR_ROLL_MODE_THRESHOLD", "Descriptive Name"="Roll Mode Threshold", "Data Type"=0, "Command"="TIM:ROLL:MTIM", "Access"=2, "Range Table"="rsscope_rngRollModeThreshold", "Read Callback"="", "Write Callback"="", "Supported Models"="", "Instrument Options"="", "Flags"=0, "Help"="The roll mode is enabled automatically if the acquisition time exceeds the given value, and if TIMebase:ROLL:ENABle is set to AUTO.\n\nAvailable Repeated Capabilities:\nNone\n\nRemote-control command(s):\nTIMebase:ROLL:MTIMe"}, {"Level"=2, "Class Only"=FALSE, "Identifier"="RSSCOPE_ATTR_ULTRA_SEGMENTATION_ENABLED", "Descriptive Name"="Ultra Segmentation Enabled", "Data Type"=3, "Command"="ACQ:SEGM:STAT", "Access"=2, "Range Table"="", "Read Callback"="", "Write Callback"="", "Supported Models"="", "Instrument Options"="", "Flags"=0, "Help"="Switches the Ultra Segmentation mode on and off.\n\nAvailable Repeated Capabilities:\nNone\n\nRemote-control command(s):\nACQuire:SEGMented:STATe"}, {"Level"=2, "Class Only"=FALSE, "Identifier"="RSSCOPE_ATTR_ULTRA_SEGMENTATION_DEPENDENCY", "Descriptive Name"="Ultra Segmentation Dependency", "Data Type"=3, "Command"="ACQ:SEGM:MAX", "Access"=2, "Range Table"="", "Read Callback"="", "Write Callback"="", "Supported Models"="", "Instrument Options"="", "Flags"=0, "Help"="The number of acquisitions in a Ultra Segmentation acquisition series depends on the record length.\n\nAvailable Repeated Capabilities:\nNone\n\nRemote-control command(s):\nACQuire:SEGMented:MAX"}, {"Level"=2, "Class Only"=FALSE, "Identifier"="RSSCOPE_ATTR_ULTRA_SEGMENTATION_AUTO_REPLAY", "Descriptive Name"="Ultra Segmentation Auto Replay", "Data Type"=3, "Command"="ACQ:SEGM:AUT", "Access"=2, "Range Table"="", "Read Callback"="", "Write Callback"="", "Supported Models"="", "Instrument Options"="", "Flags"=0, "Help"="If enabled, the instrument starts processing and displaying the data as soon as the acquisition series is captured completely. Depending on the number of acquisitions, it may take some time until the acquisition series is displayed. If the setting is disabled, the instrument only captures the data and stores it in the sample memory.\n\nAvailable Repeated Capabilities:\nNone\n\nRemote-control command(s):\nACQuire:SEGMented:AUToreplay"}, {"Level"=2, "Class Only"=FALSE, "Identifier"="RSSCOPE_ATTR_CALIBRATION_SOURCE_STATE", "Descriptive Name"="Calibration Source State", "Data Type"=3, "Command"="CAL:SOUR:STAT", "Access"=2, "Range Table"="", "Read Callback"="", "Write Callback"="", "Supported Models"="", "Instrument Options"="", "Flags"=0, "Help"="Defines the state of the internal calibration source.\n\nAvailable Repeated Capabilities:\nNone\n\nRemote-control command(s):\nCALibration:SOURce:STATe"}, {"Level"=2, "Class Only"=FALSE, "Identifier"="RSSCOPE_ATTR_CALIBRATION_SOURCE_FREQUENCY", "Descriptive Name"="Calibration Source Frequency", "Data Type"=0, "Command"="CAL:SOUR:FREQ", "Access"=2, "Range Table"="rsscope_rngCalibrationSourceFrequency", "Read Callback"="", "Write Callback"="", "Supported Models"="", "Instrument Options"="", "Flags"=0, "Help"="Frequency value of the internal calibration source. Possible values are a 1 GHz sine wave or a 10 MHz square wave.\n\nAvailable Repeated Capabilities:\nNone\n\nRemote-control command(s):\nCALibration:SOURce:FREQuency"}, {"Level"=2, "Class Only"=FALSE, "Identifier"="RSSCOPE_ATTR_CALIBRATION_OPERATING_MODE", "Descriptive Name"="Calibration Operating Mode", "Data Type"=0, "Command"="CAL:SOUR:MODE", "Access"=2, "Range Table"="rsscope_rngCalibrationOperatingMode", "Read Callback"="", "Write Callback"="", "Supported Models"="", "Instrument Options"="", "Flags"=0, "Help"="Sets the calibration operating mode. To determine the skew offset, use the &apos;Skew&apos; operating mode. It uses the internal channel alignment for best results.\n\nAvailable Repeated Capabilities:\nNone\n\nRemote-control command(s):\nCALibration:SOURce:MODE"}, {"Level"=2, "Class Only"=FALSE, "Identifier"="RSSCOPE_ATTR_CALIBRATION_DESTINATION", "Descriptive Name"="Calibration Destination", "Data Type"=0, "Command"="CAL:SOUR:SKEW:DEST", "Access"=2, "Range Table"="rsscope_rngCalibrationDestination", "Read Callback"="", "Write Callback"="", "Supported Models"="", "Instrument Options"="", "Flags"=0, "Help"="Sets the output for the calbration signal.\n\nAvailable Repeated Capabilities:\nNone\n\nRemote-control command(s):\nCALibration:SOURce:SKEW:DESTination"}, {"Level"=2, "Class Only"=FALSE, "Identifier"="RSSCOPE_ATTR_CALIBRATION_RESULT", "Descriptive Name"="Calibration Result", "Data Type"=0, "Command"="CAL:RES?", "Access"=0, "Range Table"="RsScope_rngCalibrationResult", "Read Callback"="", "Write Callback"="", "Supported Models"="", "Instrument Options"="", "Flags"=0, "Help"="Returns the result of the last selfalignment and the current alignment status. In remote mode, *CAL? provides more detailed information.\n\nAvailable Repeated Capabilities:\nNone\n\nRemote-control command(s):\nCALibration:RESult?"}, {"Level"=2, "Class Only"=FALSE, "Identifier"="RSSCOPE_ATTR_CALIBRATION_DATE", "Descriptive Name"="Calibration Date", "Data Type"=2, "Command"="CAL:DATE?", "Access"=0, "Range Table"="", "Read Callback"="", "Write Callback"="", "Supported Models"="", "Instrument Options"="", "Flags"=0, "Help"="Returns the date of the last selfalignment.\n\nAvailable Repeated Capabilities:\nNone\n\nRemote-control command(s):\nCALibration:DATE?"}, {"Level"=2, "Class Only"=FALSE, "Identifier"="RSSCOPE_ATTR_CALIBRATION_TIME", "Descriptive Name"="Calibration Time", "Data Type"=2, "Command"="CAL:TIME?", "Access"=0, "Range Table"="", "Read Callback"="", "Write Callback"="", "Supported Models"="", "Instrument Options"="", "Flags"=0, "Help"="Returns the time of the last selfalignment.\n\nAvailable Repeated Capabilities:\nNone\n\nRemote-control command(s):\nCALibration:TIME?"}, {"Level"=2, "Class Only"=FALSE, "Identifier"="RSSCOPE_ATTR_REF_OSCILLATOR_SOURCE", "Descriptive Name"="Ref Oscillator Source", 
